vi "Rising Edge Detect.vi"(4 "Input":bool) -> (1 "Pulse":bool)   [LabVIEW 2013, in "IRIO.lvlib"]
doc: "This VI generates a single-cycle pulse each time there is a low-to-high transition on the input signal. This makes it easy to detect rising edges on signals."
uses:
  IRIO.lvlib
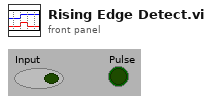
[diagram p1: front panel]
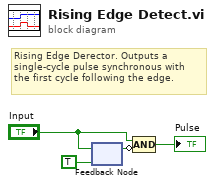
[diagram p0: block diagram]
diagram:
  # "Rising Edge Derector. Outputs a\nsingle-cycle pulse synchronous with\nthe first cycle following the edge."
  n1 = feedback-in #1("Input") -> ()
  n2 = feedback #1(TRUE ("FV")) -> (w3:bool)
  n3 = Compound Arithmetic op=AND("Input", invert w3) -> (→"Pulse":bool)
